vi "base64url Decode.vi"(11 "Base64url (or Base64)":string) -> (3 "Decoded":string)   [LabVIEW 2020, in "Base64 Support.lvlib"]
uses:
  <vilib>/JDP Science/JSONtext/Base64/Base64 Support.lvlib
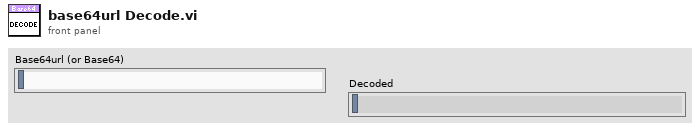
[diagram p1: front panel]
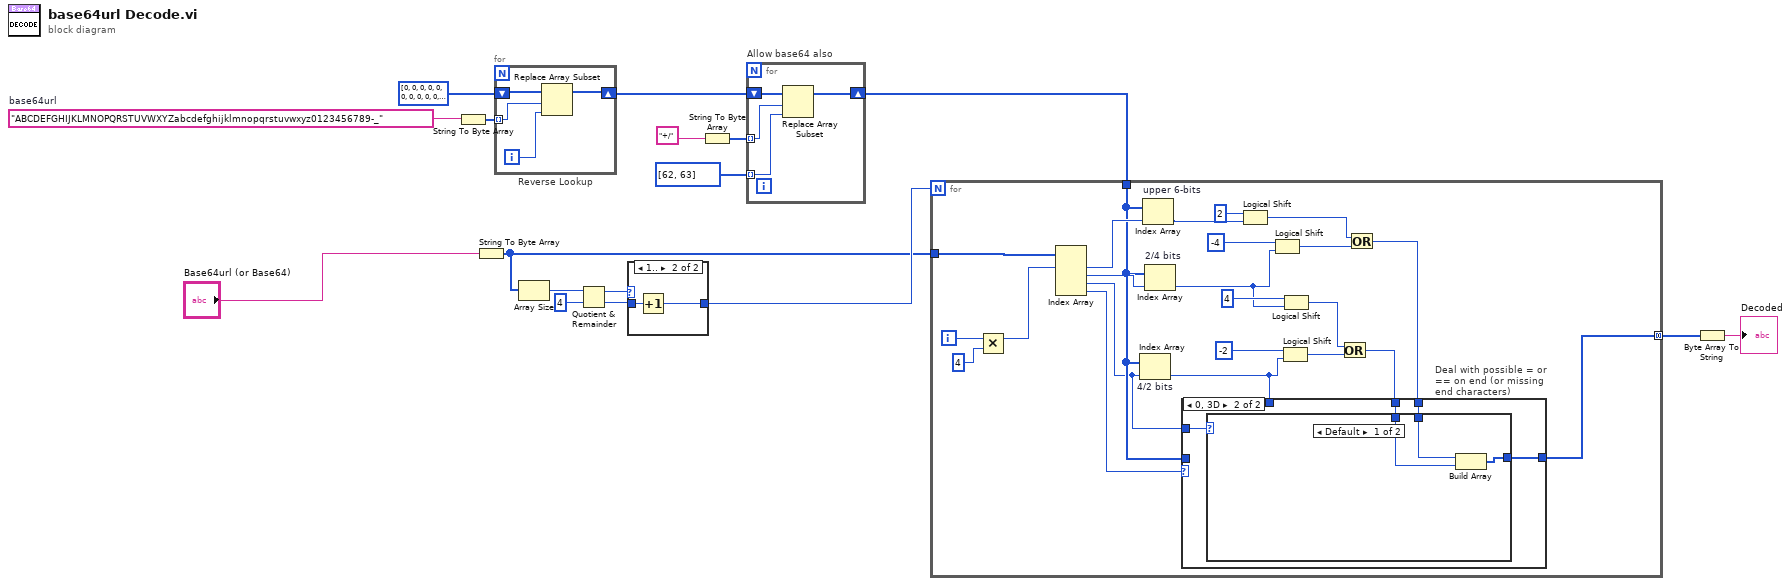
[diagram p0: block diagram]
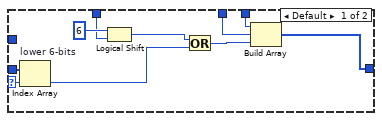
[diagram p2: hidden frame]
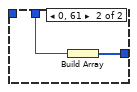
[diagram p3: hidden frame]
diagram:
  w13 = "ABCDEFGHIJKLMNOPQRSTUVWXYZabcdefghijklmnopqrstuvwxyz0123456789-_"  # base64url
  n1 = String To Byte Array(string=w13) -> (unsigned byte array=w12:u8[])
  n2 = String To Byte Array(string="Base64url (or Base64)") -> (unsigned byte array=w10:u8[])
  n3 = for "Reverse Lookup" {
    tunnel: w12 -> [w19] mode=indexing
    shift-right: [w20] -> w9
    shift-left: u8[] [0, 0, 0, 0, 0, 0, 0, 0, 0, 0, 0, 0, 0, 0, 0, 0, 0, 0, 0, 0, 0, 0, 0, 0, 0, 0, 0, 0, 0, 0, 0, 0, 0, 0, 0, 0, 0, 0, 0, 0, 0, 0, 0, 0, 0, 0, 0, 0, 0, 0, 0, 0, 0, 0, 0, 0, 0, 0, 0, 0, 0, 0, 0, 0, 0, 0, 0, 0, 0, 0, 0, 0, 0, 0, 0, 0, 0, 0, 0, 0, 0, 0, 0, 0, 0, 0, 0, 0, 0, 0, 0, 0, 0, 0, 0, 0, 0, 0, 0, 0, 0, 0, 0, 0, 0, 0, 0, 0, 0, 0, 0, 0, 0, 0, 0, 0, 0, 0, 0, 0, 0, 0, 0, 0, 0, 0, 0, 0] ("unsigned byte array") -> [w21]
    i -> [w18]
    n4 = Replace Array Subset(array=w21, new element=w18, index=w19) -> (w20:u8[])
  }
  n5 = Array Size(array=w10) -> (size(s)=w17:i32)
  n6 = Quotient & Remainder(x=w17, y=4) -> (x-y*floor(x/y)=w3:i32, floor(x/y)=w15:i32)
  n7 = case shown="1.." w3 {
    tunnel: w15 -> [w22 w24]
    tunnel: [w22 w23] -> w14
    frame ..0 {
    }
    frame 1.. {
      n8 = Increment(x=w24) -> (x+1=w23:i32)
    }
  }
  n9 = String To Byte Array(string="+/" ("String")) -> (unsigned byte array=w7:u8[])
  n10 = for "Allow base64 also" {
    shift-right: [w27] -> w5
    shift-left: w9 -> [w28]
    tunnel: w7 -> [w26] mode=indexing
    tunnel: u8[] [62, 63] ("unsigned byte array") -> [w25] mode=indexing
    n11 = Replace Array Subset(array=w28, new element=w25, index=w26) -> (w27:u8[])
  }
  n12 = for {
    N: w14 -> [_]
    tunnel: w10 -> [w51]
    tunnel: w5 -> [w47]
    tunnel: [w29] -> w4 mode=concatenating
    i -> [w50]
    n13 = Multiply(x=w50, y=4) -> (x*y=w45:i32)
    n14 = Index Array(array=w51, index #1=w45) -> (element #1=w49:u8, element #2=w48:u8, element #3=w30:u8, element #4=w46:u8)  [unwired: 3 in]
    n15 = Index Array "4/2 bits"(array=w47, index=w30) -> (element=w34:u8)
    n16 = Index Array "upper 6-bits"(array=w47, index=w49) -> (element=w42:u8)
    n17 = Index Array "2/4 bits"(array=w47, index=w48) -> (element=w37:u8)
    n18 = Logical Shift(y=i16 2, x=w42) -> (x << y=w40:u8)
    n19 = Logical Shift(y=i16 -4, x=w37) -> (x << y=w36:u8)
    n20 = Logical Shift(y=i16 -2, x=w34) -> (x << y=w32:u8)
    n21 = Logical Shift(y=i16 4, x=w37) -> (x << y=w33:u8)
    n22 = Or(x=w33, y=w32) -> (x .or. y?=w31:u8)
    n23 = Or(x=w40, y=w36) -> (x .or. y?=w39:u8)
    n24 = case "Deal with possible = or == on end (or missing end characters)" shown="0, 3D" w46 {
      selector: w46 -> [w60 _]
      tunnel: w47 -> [w61 _]
      tunnel: w39 -> [w59 w64]
      tunnel: w34 -> [w54 _]
      tunnel: w31 -> [w53 w62]
      tunnel: w30 -> [_ w65]
      tunnel: [w52 w63] -> w29
      frame Default {
        n25 = Index Array "lower 6-bits"(array=w61, index=w60) -> (element=w57:u8)
        n26 = Logical Shift(y=i16 6, x=w54) -> (x << y=w56:u8)
        n27 = Or(x=w56, y=w57) -> (x .or. y?=w55:u8)
        n28 = Build Array(w59, w53, w55) -> (w52:u8[])
      }
      frame 0, 61 {
        n29 = case shown="Default" w65 {
          tunnel: w64 -> [w68 w70]
          tunnel: [w67 w69] -> w63
          tunnel: w62 -> [w66 _]
          frame Default {
            n30 = Build Array(w68, w66) -> (w67:u8[])
          }
          frame 0, 61 {
            n31 = Build Array(w70) -> (w69:u8[])
          }
        }
      }
    }
  }
  n32 = Byte Array To String(unsigned byte array=w4) -> (string=→"Decoded":string)
